vi "AnyBuilderBegin.vi"(7 "error in":errorcluster) -> (0 "error out":errorcluster, 3 "Builder Ref Out":T1)   [LabVIEW 2019, in "grpc-lvsupport.lvlib"]
uses:
  grpc-lvsupport.lvlib
  grpcId.ctl
  <vilib>/Utility/error.llb/Error Cluster From Error Code.vi
  <resource>/libgrpc_labview.dll
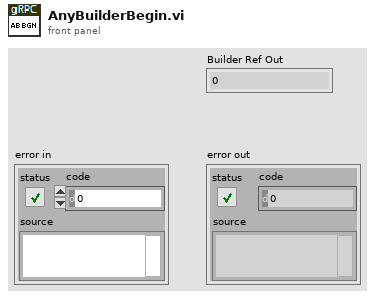
[diagram p1: front panel]
types:
  T1 = typedef "grpc-lvsupport.lvlib/grpcId.ctl" = u64
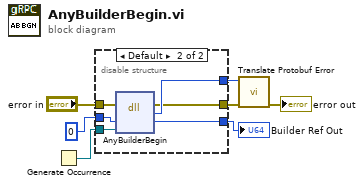
[diagram p0: block diagram]
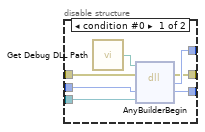
[diagram p2: hidden frame]
diagram:
  n1 = Generate Occurrence() -> (w1:refnum<k4>)
  n2 = disable-structure shown="Default" {
    disable-tunnel: [w13 w20] -> w7
    disable-tunnel: [w12 w19] -> w6
    disable-tunnel: w1 -> [w11 w18]
    disable-tunnel: "error in" -> [w10 w17]
    disable-tunnel: [w9 w16] -> w5
    disable-tunnel: u64 0 ("anyId") -> [w8 w15]
    frame condition #0 {
      n3 = call "Get Debug DLL Path.vi"() -> ("DLL Path"=w14:path)
      n4 = dll-call lib="?" fn="AnyBuilderBegin"(path in=w14, error in=w10, "anyId"=w8, "InitCallbacksOccurrence"=w11) -> (error out=w9:errorcluster, "return type"=w12:i32, "anyId"=w13:u64)  [unwired: 2 in, 1 out]
    }
    frame condition #1 (active) {
      n5 = dll-call lib="C:/Program Files (x86)/National Instruments/LabVIEW 2024/resource/libgrpc_labview.*" fn="AnyBuilderBegin"(error in=w17, "anyId"=w15, "InitCallbacksOccurrence"=w18) -> (error out=w16:errorcluster, "return type"=w19:i32, "anyId"=w20:u64)  [unwired: 3 in, 1 out]
    }
  }
  "Builder Ref Out" <- w7
  n6 = call "Translate Protobuf Error.vi"("error in"=w5, "Error Code"=w6) -> ("error out"=→"error out":errorcluster)  [unwired: 9 in]
